vi "2D Helmholtz PDE Solver (Polygon Domain).vi"(0 "PDE in":refnum<class "NI_PDE.lvclass">, 11 "error in (no error)":errorcluster) -> (4 "PDE out":refnum<class "NI_PDE.lvclass">, 6 "U(x, y)":dbl[](array[numeric]), 8 "Grid Points":cluster{"X":dbl, "Y":dbl}[](array[cluster]), 15 "error out":errorcluster)   [LabVIEW 2020, in "NI_PDE.lvlib"]
doc: "Solves a partial differential equation. You must manually select the polymorphic instance to use."
uses:
  <vilib>/gmath/NI_PDE.lvlib
  <vilib>/gmath/pde.llb/PDEClass/NI_PDE.lvclass
  <vilib>/gmath/pde.llb/PDEClass/PDE_Helmholtz_2D/NI_PDE_Helmholtz_2D.lvclass
  e:/builds/penguin/labview/branches/2020/dev/dist/vi.lib/gmath/pde.llb/PDEClass/NI_PDE.lvclass
  <vilib>/gmath/pde.llb/DomainClass/Domain_Steady_2D_Polygon/NI_Domain_Steady_2D_Polygon.lvclass
  e:/builds/penguin/labview/branches/2020/dev/dist/vi.lib/gmath/pde.llb/DomainClass/NI_Domain.lvclass
  <vilib>/gmath/pde.llb/RHSClass/RHS_2D_Numeric/NI_RHS_2D_Numeric.lvclass
  e:/builds/penguin/labview/branches/2020/dev/dist/vi.lib/gmath/pde.llb/RHSClass/NI_RHS.lvclass
  <vilib>/gmath/pde.llb/BCClass/BC_Steady_2D_Numeric/NI_BC_Steady_2D_Numeric.lvclass
  e:/builds/penguin/labview/branches/2020/dev/dist/vi.lib/gmath/pde.llb/BCClass/NI_BC.lvclass
  <vilib>/gmath/pde.llb/PDEClass/PDE_2ndOrder_ConstPara/Para Data.ctl
  <vilib>/gmath/pde.llb/PDEClass/PDE Data_Class.ctl
  <vilib>/gmath/pde.llb/RHSClass/NI_RHS.lvclass
  <vilib>/gmath/pde.llb/DomainClass/NI_Domain.lvclass
  <vilib>/gmath/pde.llb/BCClass/NI_BC.lvclass
  <vilib>/gmath/pde.llb/ICClass/NI_IC.lvclass
  <vilib>/gmath/pde.llb/BCClass/BC_Steady_2D_Numeric/BC Data.ctl
  <vilib>/gmath/pde.llb/Common/PDE_BC Type.ctl
  <vilib>/gmath/pde.llb/Common/PDE_BC Position 2D.ctl
  <vilib>/gmath/pde.llb/DomainClass/Domain_Steady_2D_Polygon/Domain Data.ctl
  <vilib>/gmath/pde.llb/PDEClass/PDE_2ndOrder_ConstPara/NI_PDE_2ndOrder_ConstPara.lvclass
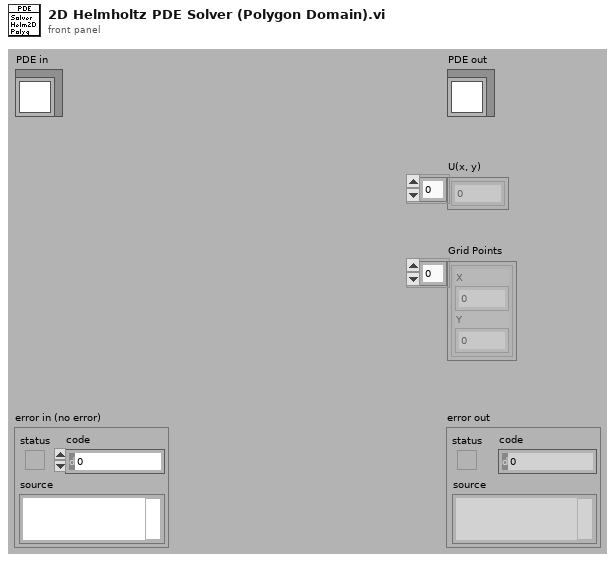
[diagram p1: front panel]
types:
  T1 = typedef "NI_PDE.lvlib/NI_Domain_Steady_2D_Polygon.lvclass/Domain Data.ctl" = cluster{"X":dbl[], "Y":dbl[], "Xi":dbl[], "Yi":dbl[], "grid factor":dbl, "Triangulation":i32[][]}
  T2 = typedef "NI_PDE.lvlib/NI_BC_Steady_2D_Numeric.lvclass/BC Data.ctl" = cluster{"type":T3, "position":T4, "G":dbl[]}
  T3 = typedef "NI_PDE.lvlib/PDE_BC Type.ctl" = i32
  T4 = typedef "NI_PDE.lvlib/PDE_BC Position 2D.ctl" = i32
  T5 = typedef "NI_PDE.lvlib/NI_PDE.lvclass/PDE Data_Class.ctl" = cluster{"PDE":refnum<class "NI_PDE.lvclass">, "RHS":refnum<class "NI_RHS.lvclass">, "Domain":refnum<class "NI_Domain.lvclass">, "BC":refnum<class "NI_BC.lvclass">, "IC":refnum<class "NI_IC.lvclass">}
  T6 = typedef "NI_PDE.lvlib/NI_PDE_2ndOrder_ConstPara.lvclass/Para Data.ctl" = cluster{"k":dbl, "a":dbl}
  T7 = typedef "NI_PDE.lvlib/NI_PDE.lvclass/PDE Data_Variant.ctl" = cluster{"parameter":variant, "RHS":variant, "domain":variant, "BC Array":variant[], "IC Array":variant[]}
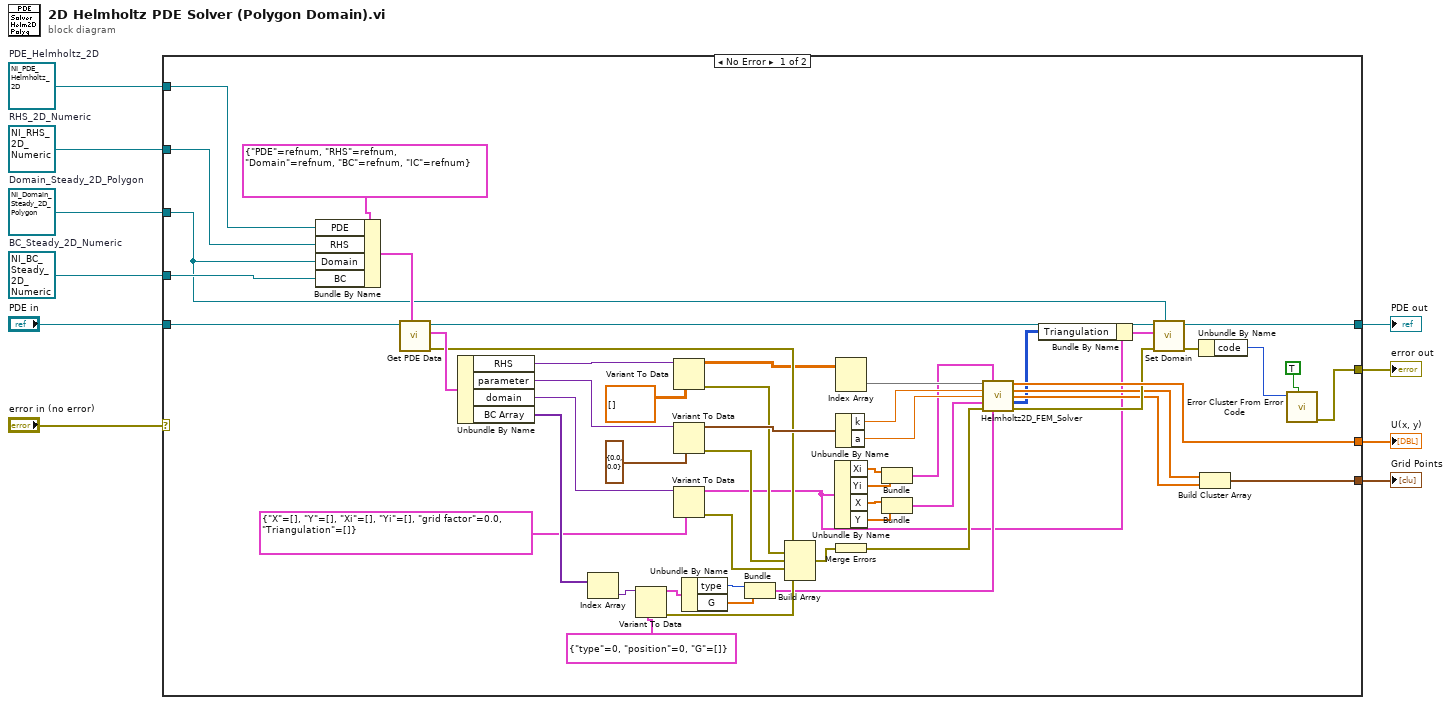
[diagram p0: block diagram]
diagram:
  w1 = refnum<class "NI_BC_Steady_2D_Numeric.lvclass"> refnum  # BC_Steady_2D_Numeric
  w2 = refnum<class "NI_RHS_2D_Numeric.lvclass"> refnum  # RHS_2D_Numeric
  w3 = refnum<class "NI_Domain_Steady_2D_Polygon.lvclass"> refnum  # Domain_Steady_2D_Polygon
  w4 = refnum<class "NI_PDE_Helmholtz_2D.lvclass"> refnum  # PDE_Helmholtz_2D
  n1 = case shown="No Error" "error in (no error)" {
    selector: "error in (no error)" -> [_ w65]
    tunnel: "PDE in" -> [w37 w64]
    tunnel: [w63 _] -> w9
    tunnel: [w62 w64] -> w8
    tunnel: [w58 _] -> w7
    tunnel: [w54 w65] -> w6
    tunnel: w4 -> [w18 _]
    tunnel: w2 -> [w17 _]
    tunnel: w3 -> [w12 _]
    tunnel: w1 -> [w16 _]
    frame No Error {
      n2 = Bundle By Name(cluster=T5 {"PDE"=refnum, "RHS"=refnum, "Domain"=refnum, "BC"=refnum, "IC"=refnum} ("target class"), "PDE"=w18, "RHS"=w17, "Domain"=w12, "BC"=w16) -> (w39:T5)
      n3 = call <vilib>:"Get PDE Data.vi"("target class"=w39, "PDE in"=w37) -> ("error out"=w41:errorcluster, "PDE data"=w45:T7, "PDE out"=w38:refnum<class "NI_PDE.lvclass">)  [unwired: 3 in, 4 out]
      n4 = Unbundle By Name(w45) -> ("RHS"=w43:variant, "parameter"=w44:variant, "domain"=w42:variant, "BC Array"=w32:variant[])
      n5 = Index Array(array=w32) -> (element=w31:variant)  [unwired: 1 in]
      n6 = Variant To Data(type=T2 {"type"=0, "position"=0, "G"=[]} ("BC data"), Variant=w31) -> (data=w36:T2, error out=w47:errorcluster)  [unwired: 1 in]
      n7 = Variant To Data(type=dbl[][] [] ("F(x, y)"), Variant=w43) -> (data=w23:dbl[][], error out=w50:errorcluster)  [unwired: 1 in]
      n8 = Variant To Data(type=T6 {"k"=0.0, "a"=0.0} ("para data"), Variant=w44) -> (data=w52:T6, error out=w49:errorcluster)  [unwired: 1 in]
      n9 = Variant To Data(type=T1 {"X"=[], "Y"=[], "Xi"=[], "Yi"=[], "grid factor"=0.0, "Triangulation"=[]} ("domain data"), Variant=w42) -> (data=w11:T1, error out=w48:errorcluster)  [unwired: 1 in]
      n10 = Unbundle By Name(w36) -> ("type"=w35:T3, "G"=w34:dbl[])
      n11 = Bundle("type"=w35, "G"=w34) -> (w30:cluster{"type":T3, "G":dbl[]})  [unwired: 1 out]
      n12 = Build Array(w41, w50, w49, w48, w47) -> (w46:errorcluster[])
      n13 = Unbundle By Name(w11) -> ("Xi"=w21:dbl[], "Yi"=w20:dbl[], "X"=w28:dbl[], "Y"=w27:dbl[])
      n14 = Index Array(array=w23) -> (element=w22:dbl[])  [unwired: 2 in]
      n15 = Unbundle By Name(w52) -> ("k"=w25:dbl, "a"=w24:dbl)
      n16 = Merge Errors(w46) -> (w29:errorcluster)
      n17 = Bundle("Xi"=w21, "Yi"=w20) -> (w19:cluster{"Xi":dbl[], "Yi":dbl[]})  [unwired: 1 out]
      n18 = Bundle("X"=w28, "Y"=w27) -> (w26:cluster{"X":dbl[], "Y":dbl[]})  [unwired: 1 out]
      n19 = call <vilib>:"Helmholtz2D_FEM_Solver.vi"("F(x, y)"=w22, "Grid"=w19, "k"=w25, "a"=w24, "Domain"=w26, "error in (no error)"=w29, "Boundary Condition"=w30) -> ("U(x, y)"=w63:dbl[], "X Used"=w60:dbl[], "Y Used"=w59:dbl[], "Triangulation"=w15:i32[][], "error out"=w61:errorcluster)  [unwired: 1 in, 3 out]
      n20 = Bundle By Name(cluster=w11, "Triangulation"=w15) -> (w14:T1)
      n21 = call <vilib>:"Set Domain.vi"("target Domain"=w12, "error in (no error)"=w61, "domain"=w14, "PDE in"=w38) -> ("error out"=w55:errorcluster, "PDE out"=w62:refnum<class "NI_PDE.lvclass">)  [unwired: 6 out]
      n22 = Unbundle By Name(w55) -> ("code"=w57:i32)
      n23 = Build Cluster Array(w60, w59) -> (w58:cluster{"Numeric":dbl, "Numeric":dbl}[])
      n24 = call <vilib>:"Error Cluster From Error Code.vi"("show call chain? (False)"=TRUE, "error code (0)"=w57) -> ("error out"=w54:errorcluster)  [unwired: 1 in, 6 out]
    }
    frame Error {
    }
  }
  "U(x, y)" <- w9
  "error out" <- w6
  "PDE out" <- w8
  "Grid Points" <- w7
